vi "New Connection.vi"(8 "error in (no error)":errorcluster, 10 "Socket":refnum<class "Socket.lvclass">, 11 "Connection Listener in":refnum<class "Connection Listener.lvclass">) -> (0 "error out":errorcluster, 3 "Connection Listener out":refnum<class "Connection Listener.lvclass">)   [LabVIEW 2017, in "Connection Listener.lvlib" / "Connection Listener.lvclass"]
uses:
  Connection Listener.lvclass
  Applications/National Instruments/LabVIEW 2017 64-bit/vi.lib/ActorFramework/Actor/Actor.lvclass
  <vilib>/MediaMongrels Ltd/WebSockets/Sockets/Socket/Socket.lvclass
  Connection Listener.lvclass/Connection Listener.ctl
  Get Next ID.vi
  Connection Handler/Connection Handler/Connection Handler.lvclass
  <vilib>/ActorFramework/Actor/Actor.lvclass
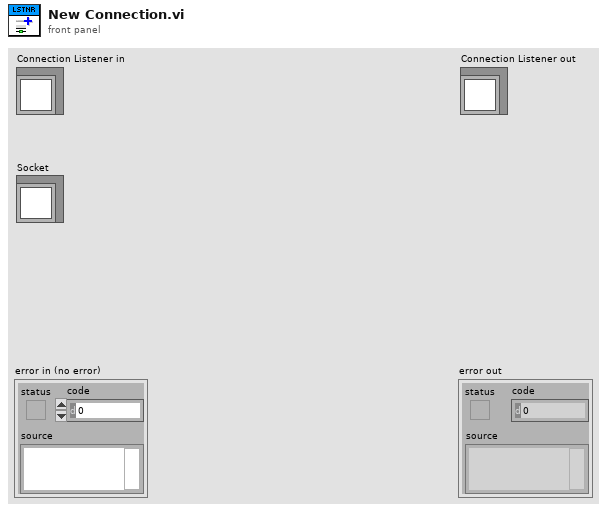
[diagram p1: front panel]
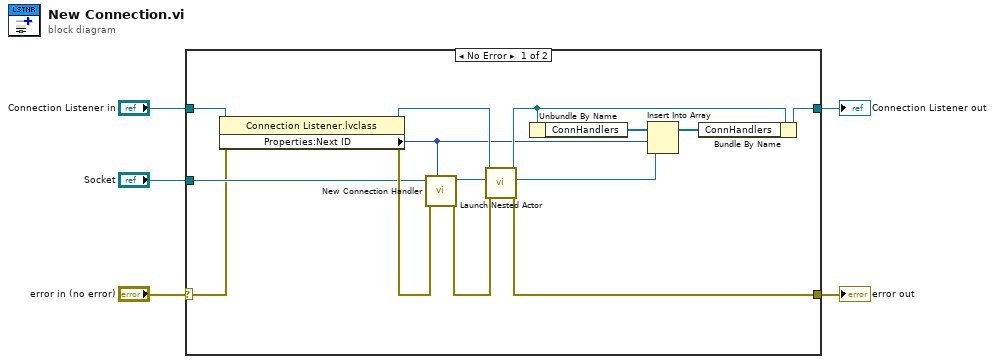
[diagram p0: block diagram]
diagram:
  n1 = case shown="No Error" "error in (no error)" {
    selector: "error in (no error)" -> [w6 w21]
    tunnel: [w16 w21] -> w4
    tunnel: [w14 w20] -> w2
    tunnel: "Connection Listener in" -> [w18 w20]
    tunnel: "Socket" -> [w7 _]
    frame No Error {
      n2 = property class="Connection Listener.lvclass"(reference=w18, error in=w6) -> (reference out=w15:refnum<class "Connection Listener.lvclass">, error out=w8:errorcluster, "Properties:Next ID"=w9:i32)
      n3 = call "New Connection Handler.vi"("ID"=w9, "error in (no error)"=w8, "Socket"=w7) -> ("error out"=w17:errorcluster, "Connection Handler out"=w19:refnum<class "Connection Handler.lvclass">)  [unwired: 7 in]
      n4 = call <vilib>:"Launch Nested Actor.vi"("error in (no error)"=w17, "Nested Actor"=w19, "Caller Actor in"=w15) -> ("error out"=w16:errorcluster, "Nested Actor's Enqueuer"=w10:refnum<class "Message Enqueuer.lvclass">, "Caller Actor out"=w13:refnum<class "Connection Listener.lvclass">)  [unwired: 6 in]
      n5 = Unbundle By Name(w13) -> ("ConnHandlers"=w12:refnum<class "Message Enqueuer.lvclass">[])
      n6 = Insert Into Array(array=w12, index=w9, new element=w10) -> (w11:refnum<class "Message Enqueuer.lvclass">[])
      n7 = Bundle By Name(cluster=w13, "ConnHandlers"=w11) -> (w14:refnum<class "Connection Listener.lvclass">)
    }
    frame Error {
    }
  }
  "error out" <- w4
  "Connection Listener out" <- w2
